vi "Photodetector DAQ.vi"() -> ()   [LabVIEW 2018]
uses:
  Documents/GitHub/electrostatic-lens-labview-controller/Sub VIs/Save data to file (double).vi
panel:
  in  "Save data?":bool caption="Enable"
  in  "Save data path":path
  in  "stop":bool
  out "PMT":dynamicdata(graph)
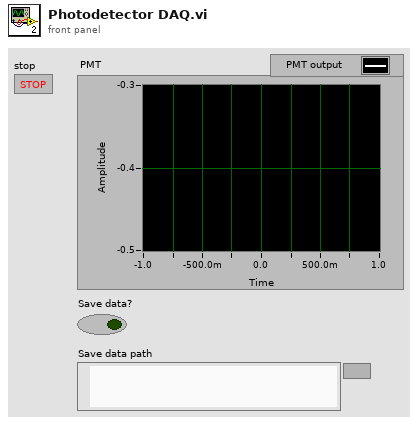
[diagram p1: front panel]
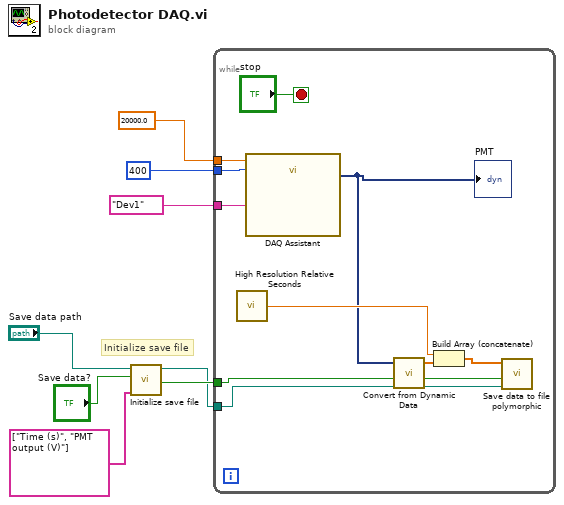
[diagram p0: block diagram]
diagram:
  # "Initialize save file"
  n1 = call "Initialize save file.vi"("Array"=string[] ["Time (s)", "PMT output (V)"], "Save data? in"="Save data?", "Save data path in"="Save data path") -> ("Save data? out"=w3:bool, "Save data path out"=w2:path)  [unwired: 7 in]
  n2 = while {
    tunnel: tag "Dev1" ("device name") -> [w18]
    tunnel: 20000.0 ("rate") -> [w17]
    tunnel: 400 ("number of samples") -> [w15]
    tunnel: w3 -> [w14]
    tunnel: w2 -> [w13]
    stop <- "stop" stop-if-true
    n3 = call <vilib>:"High Resolution Relative Seconds.vi"() -> ("relative seconds"=w10:dbl)
    n4 = call "DAQ Assistant"("rate"=w17, "number of samples"=w15, "device name"=w18) -> ("data"=w9:dynamicdata)  [unwired: 13 in, 3 out]
    "PMT" <- w9
    n5 = call "Convert from Dynamic Data"("Dynamic Data Type"=w9) -> ("Array"=w12:dbl[])  [unwired: 3 in]
    n6 = Build Array (concatenate)(w10, w12) -> (w11:dbl[])
    n7 = call-poly "Save data to file polymorphic.vi"("File path"=w13, "Save data?"=w14, "Data"=w11) -> ()  [unwired: 9 in]
  }
